vi "BKPrecPractice.vi"() -> ()   [LabVIEW 2023]
uses:
  <vilib>/DAQmx/read.llb/DAQmx Read (Analog DBL 1Chan 1Samp).vi
  <vilib>/DAQmx/create/channels.llb/DAQmx Create Channel (AI-Voltage-Basic).vi
  <vilib>/DAQmx/configure/timing.llb/DAQmx Timing (Sample Clock).vi
  <vilib>/DAQmx/configure/events/hardwareSignals.llb/DAQmx Export Signal (Most Signals).vi
  <vilib>/DAQmx/miscellaneous.llb/DAQmx Fill In Error Info.vi
  <instrlib>/BK Precision 4050 Series/BK Precision 4050 Series.lvlib
panel:
  out "Waveform Chart":dbl(graph)
  in  "Database Square":bool
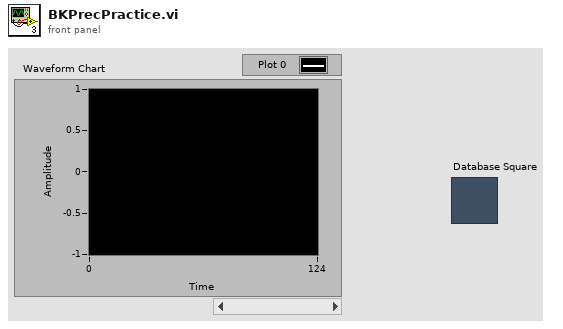
[diagram p1: front panel]
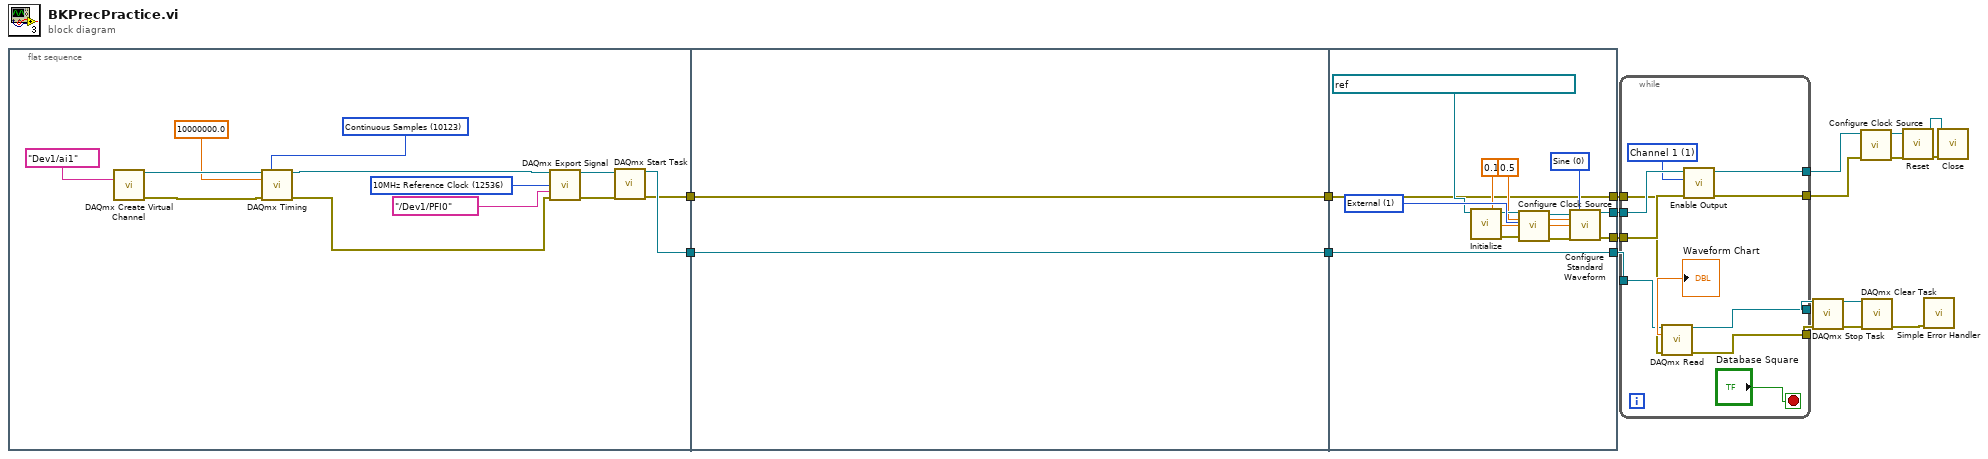
[diagram p0: block diagram]
diagram:
  n1 = flat-sequence {
    tunnel: [w27] -> w5
    tunnel: [w21] -> w1
    tunnel: w5 -> [w34]
    tunnel: [w34] -> w4
    tunnel: [w33] -> w2
    tunnel: w1 -> [w33]
    tunnel: [w36] -> w14
    tunnel: [w38] -> w13
    tunnel: [w37] -> w12
    tunnel: w4 -> [w36]
    tunnel: [w35] -> w3
    tunnel: w2 -> [w35]
    frame #0 {
      w20 = 10123 items=["Finite Samples"=10178, "Continuous Samples"=10123, "Hardware Timed Single Point"=12522] ("sample mode")
      w32 = 12536 items=["AI Convert Clock"=12484, "10MHz Reference Clock"=12536, "20MHz Timebase Clock"=12486, "Sample Clock"=12487, "Advance Trigger"=12488, "Reference Trigger"=12490, "Start Trigger"=12491, "Advance Complete Event"=12492, "AI Hold Complete Event"=12493, "Counter Output Event"=12494, "Change Detection Event"=12511, "Watchdog Timer Expired Event"=12512] ("signal")
      n2 = call-poly <vilib>:"DAQmx Create Virtual Channel.vi"("physical channels"=tag "Dev1/ai1") -> ("task out"=w23:refnum<k21>, "error out"=w26:errorcluster)  [unwired: 13 in]
      n3 = call-poly <vilib>:"DAQmx Timing.vi"("task/channels in"=w23, "sample mode"=w20, "rate"=10000000.0, "error in"=w26) -> ("task out"=w24:refnum<k21>, "error out"=w25:errorcluster)  [unwired: 10 in]
      n4 = call-poly <vilib>:"DAQmx Export Signal.vi"("task/channels in"=w24, "signal"=w32, "output terminal"=tag "/Dev1/PFI0", "error in"=w25) -> ("task out"=w29:refnum<k21>, "error out"=w28:errorcluster)  [unwired: 10 in]
      n5 = call <vilib>:"DAQmx Start Task.vi"("task/channels in"=w29, "error in"=w28) -> ("task out"=w27:refnum<k21>, "error out"=w21:errorcluster)  [unwired: 12 in]
    }
    frame #1 {
    }
    frame #2 {
      w41 = u16 0 items=["Sine", "Square", "Ramp"] ("Waveform Function (0: Sine)")
      w47 = u16 1 items=["Internal", "External"] ("Source (0: Internal)")
      n6 = call <instrlib>:"Initialize.vi"("VISA resource name"=refnum<visa-resource-name> "USB0::0xF4ED::0xEE3A::389H14130::INSTR") -> ("error out"=w44:errorcluster, "VISA resource name out"=w45:refnum<visa-resource-name>)  [unwired: 9 in]
      n7 = call <instrlib>:"Configure Clock Source.vi"("error in (no error)"=w44, "Source (0: Internal)"=w47, "VISA resource name"=w45) -> ("error out"=w42:errorcluster, "VISA resource name out"=w43:refnum<visa-resource-name>)  [unwired: 7 in]
      n8 = call <instrlib>:"Configure Standard Waveform.vi"("VISA resource name"=w43, "Waveform Function (0: Sine)"=w41, "Amplitude (1.0 Vpp)"=0.5, "Frequency (1000 Hz)"=0.1, "error in (no error)"=w42) -> ("VISA resource name out"=w38:refnum<visa-resource-name>, "error out"=w37:errorcluster)  [unwired: 9 in]
    }
  }
  n9 = while {
    tunnel: [w58] -> w19
    tunnel: [w57] -> w18
    tunnel: w14 -> [w48]
    tunnel: w13 -> [w54]
    tunnel: w12 -> [w53]
    tunnel: [w51] -> w9
    tunnel: [w50] -> w8
    tunnel: w3 -> [w49]
    stop <- "Database Square" stop-if-true
    w52 = 1 items=["Channel 1"=1, "Channel 2"=2] ("Select Channel (1:Channel 1)")
    n10 = call-poly <vilib>:"DAQmx Read.vi"("task/channels in"=w48, "error in"=w49) -> ("task out"=w58:refnum<k21>, "data"=→"Waveform Chart":dbl, "error out"=w57:errorcluster)  [unwired: 11 in]
    n11 = call <instrlib>:"Enable Output.vi"("error in (no error)"=w53, "Select Channel (1:Channel 1)"=w52, "VISA resource name"=w54) -> ("error out"=w51:errorcluster, "VISA resource name out"=w50:refnum<visa-resource-name>)  [unwired: 7 in]
  }
  n12 = call <vilib>:"DAQmx Stop Task.vi"("task/channels in"=w19, "error in"=w18) -> ("task out"=w17:refnum<k21>, "error out"=w16:errorcluster)  [unwired: 12 in]
  n13 = call <instrlib>:"Configure Clock Source.vi"("error in (no error)"=w9, "VISA resource name"=w8) -> ("error out"=w6:errorcluster, "VISA resource name out"=w7:refnum<visa-resource-name>)  [unwired: 8 in]
  n14 = call <vilib>:"DAQmx Clear Task.vi"("task in"=w17, "error in"=w16) -> ("error out"=w15:errorcluster)  [unwired: 13 in]
  n15 = call <instrlib>:"Reset.vi"("error in (no error)"=w6, "VISA resource name"=w7) -> ("error out"=w11:errorcluster, "VISA resource name out"=w10:refnum<visa-resource-name>)  [unwired: 8 in]
  n16 = call <vilib>:"Simple Error Handler.vi"("error in (no error)"=w15) -> ()  [unwired: 4 in, 5 out]
  n17 = call <instrlib>:"Close.vi"("error in (no error)"=w11, "VISA resource name"=w10) -> ()  [unwired: 9 in, 1 out]
